vi "Update System Definition Error.vi"(8 "error to report":errorcluster, 9 "error in":errorcluster, 10 "error key":string, 11 "Configuration files Ref":T1 format="%.0x") -> (0 "error out":errorcluster, 3 "Configuration files Ref out":T1 format="%.0x")   [LabVIEW 2020, in "Ballard ARINC 429 Scripting.lvlib"]
uses:
  Ballard ARINC 429 Scripting.lvlib
  <vilib>/NI VeriStand/Custom Device API/Custom Device Item Ref.ctl
  <vilib>/NI VeriStand/Custom Device API/Custom Device API.lvlib
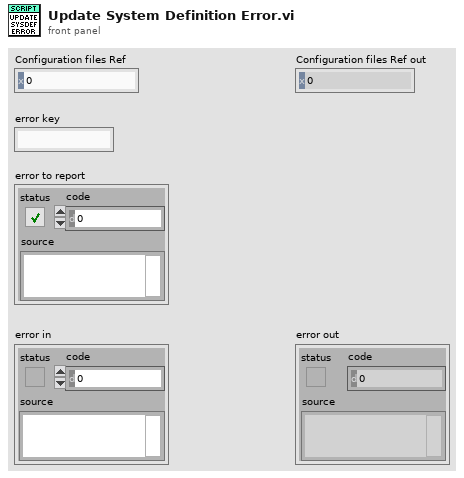
[diagram p1: front panel]
types:
  T1 = typedef "Custom Device API.lvlib/Custom Device Item Ref.ctl" = u64
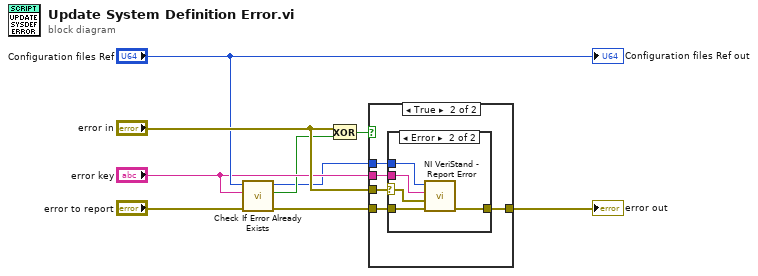
[diagram p0: block diagram]
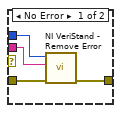
[diagram p3: hidden frame]
diagram:
  n1 = call "Check If Error Already Exists.vi"("error in"="error to report", "error key"="error key", "Configuration files Ref"="Configuration files Ref") -> ("error out"=w5:errorcluster, "error exists?"=w2:bool, "Configuration files Ref out"=w1:T1)  [unwired: 6 in]
  n2 = Exclusive Or(1:w2, 2:"error in") -> (0:w9:bool)
  n3 = case shown="True" w9 {
    tunnel: [w10 w15] -> w8
    tunnel: "error key" -> [_ w14]
    tunnel: "error in" -> [_ w13]
    tunnel: w5 -> [w10 w12]
    tunnel: w1 -> [_ w11]
    frame False {
      # "To avoid dirty dots, don't update if the error already exists."
    }
    frame True {
      n4 = case shown="Error" w13 {
        selector: w13 -> [_ w20]
        tunnel: w14 -> [w19 w24]
        tunnel: w12 -> [w17 w23]
        tunnel: [w18 w22] -> w15
        tunnel: w11 -> [w16 w21]
        frame No Error {
          n5 = call <vilib>:"NI VeriStand - Remove Error.vi"("error in (no error)"=w17, "Error ID"=w19, "Node Ref in"=w16) -> ("error out"=w18:errorcluster)  [unwired: 7 in, 1 out]
        }
        frame Error {
          n6 = call <vilib>:"NI VeriStand - Report Error.vi"("error in (no error)"=w23, "New Error"=w20, "Error ID"=w24, "Node Ref in"=w21) -> ("error out"=w22:errorcluster)  [unwired: 6 in, 1 out]
        }
      }
    }
  }
  "error out" <- w8
  "Configuration files Ref out" <- "Configuration files Ref"
